vi "align_vi_panel.vi"(8 "error in":errorcluster, 9 "ref vi reference":refnum<vi>, 10 "top vi reference":refnum<vi>, 11 "use top level VI (T)":bool=TRUE) -> (0 "error out":errorcluster)   [LabVIEW 2020, in "varilib.lvlib"]
doc: "LV does not support aligning window to parent window venter. So when this VI is called in the VI with visible panel, it aligns front panel of the caller VI to center of its parent VI front panel or top level VI front panel.\nIn case the top level VI was called asychronously it is necessary to do following:\n1) Call this VI with 'top vi reference' set to reference of the top level VI. This is typically done in main window of application.\n2) Than call this VI within the panel to align with parameter 'use top level VI' set to True. This will use the reference assigned in step 1) as a reference position.\nThis VI also has input 'ref vi reference'. This can be used to set reference position VI directly. It has priority is it is assigned."
uses:
  varilib.lvlib
panel:
  in  "top vi reference memory":refnum<vi>
  out "call chain":string[](array[string])
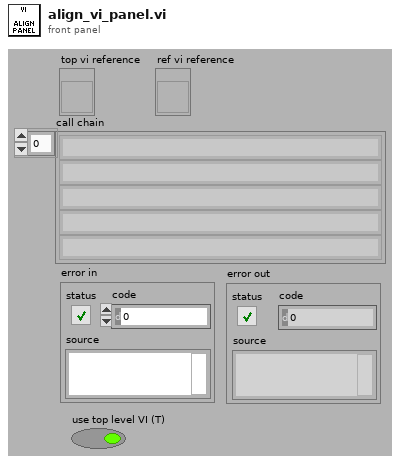
[diagram p1: front panel]
types:
  T1 = typedef "LVRectTypeDef.ctl" = cluster{"Left":i16, "Top":i16, "Right":i16, "Bottom":i16}
  T2 = enum32{"Invalid", "Standard", "Closed", "Hidden", "Minimized", "Maximized"}
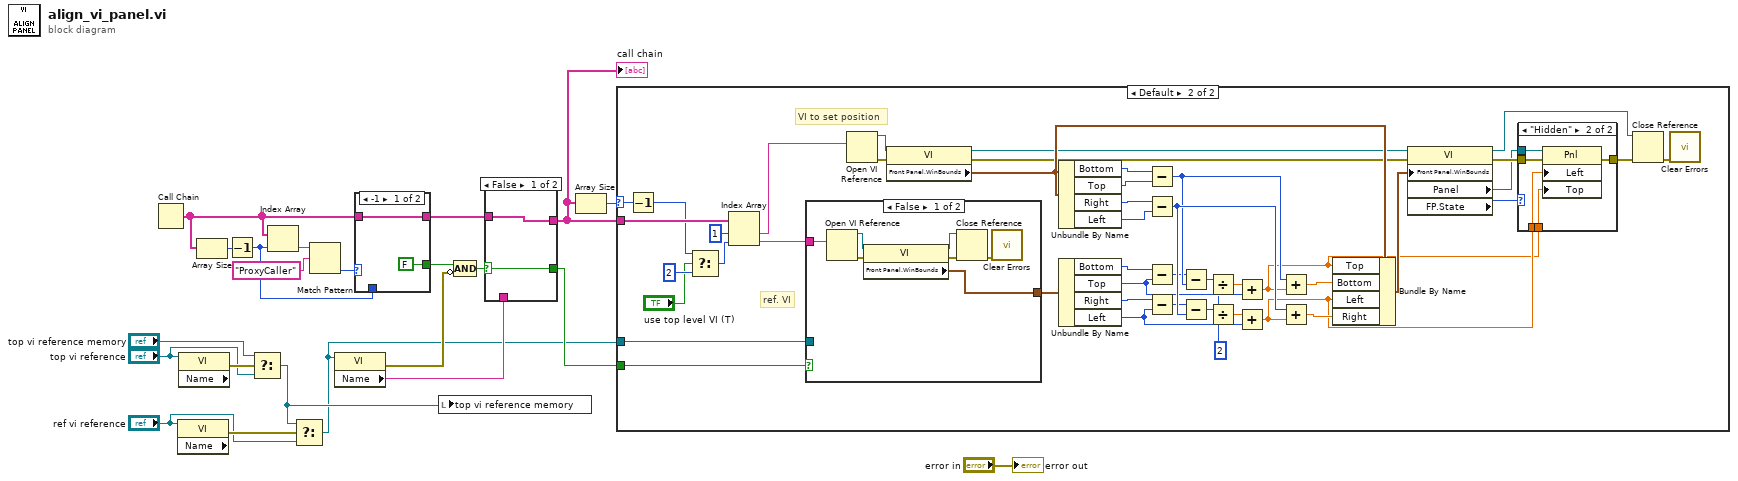
[diagram p0: block diagram]
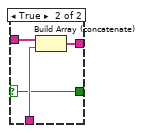
[diagram p2: hidden frame]
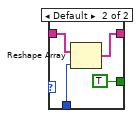
[diagram p3: hidden frame]
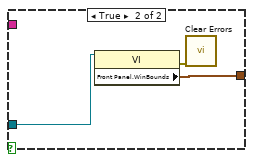
[diagram p6: hidden frame]
diagram:
  n1 = Call Chain() -> (call chain=w17:string[])
  n2 = property class="VI" props=["Name"](reference="ref vi reference") -> (error out=w4:errorcluster)  [unwired: 1 in, 2 out]
  n3 = property class="VI" props=["Name"](reference="top vi reference") -> (error out=w7:errorcluster)  [unwired: 1 in, 2 out]
  n4 = Array Size(array=w17) -> (size(s)=w20:i32)
  n5 = Decrement(x=w20) -> (x-1=w15:i32)
  n6 = Select(t="top vi reference memory", s=w7, f="top vi reference") -> (s? t:f=w2:refnum<vi>)
  n7 = Index Array(array=w17, index=w15) -> (element=w19:string)
  n8 = Select(t=w2, s=w4, f="ref vi reference") -> (s? t:f=w1:refnum<vi>)
  n9 = Match Pattern(string=w19, regular expression="ProxyCaller") -> (offset past match=w16:i32)  [unwired: 1 in, 3 out]
  n10 = property class="VI"(reference=w1) -> (error out=w8:errorcluster, "Name"=w12:string)  [unwired: 1 in, 1 out]
  n11 = case shown="-1" w16 {
    tunnel: w17 -> [w24 w28]
    tunnel: [w24 w27] -> w14
    tunnel: w15 -> [_ w26]
    tunnel: [FALSE TRUE] -> w10
    frame -1 {
    }
    frame Default {
      n12 = Reshape Array(w28, w26) -> (w27:string[])
    }
  }
  n13 = local write "top vi reference memory"(w2) -> ()
  n14 = Compound Arithmetic op=AND(w10, invert w8) -> (w11:bool)
  n15 = case shown="False" w11 {
    selector: w11 -> [w29 w31]
    tunnel: w14 -> [w30 w34]
    tunnel: [w30 w33] -> w13
    tunnel: w12 -> [_ w32]
    tunnel: [w29 w31] -> w9
    frame False {
    }
    frame True {
      n16 = Build Array (concatenate)(w34, w32) -> (w33:string[])
    }
  }
  "call chain" <- w13
  n17 = Array Size(array=w13) -> (size(s)=w21:i32)
  n18 = case shown="Default" w21 {
    selector: w21 -> [_ w48]
    tunnel: w13 -> [_ w51]
    tunnel: w1 -> [_ w43]
    tunnel: w9 -> [_ w42]
    frame 1, 2 {
    }
    frame Default {
      w71 = i16 2 ("y")
      # "ref. VI"
      # "VI to set position"
      n19 = Decrement(x=w48) -> (x-1=w47:i32)
      n20 = Select(t=w47, s="use top level VI (T)", f=2) -> (s? t:f=w49:i32)
      n21 = Index Array(array=w51, index #1=1 ("index"), index #2=w49) -> (element #1=w54:string, element #2=w44:string)
      n22 = case shown="False" w42 {
        tunnel: [w92 w95] -> w53
        tunnel: w44 -> [w86 _]
        tunnel: w43 -> [_ w94]
        frame False {
          n23 = Open VI Reference(vi path=w86) -> (vi reference=w88:refnum<vi>, error out=w89:errorcluster)  [unwired: 5 in]
          n24 = property class="VI"(reference=w88, error in=w89) -> (reference out=w91:refnum<vi>, error out=w90:errorcluster, "Front Panel.WinBounds"=w92:T1)
          n25 = Close Reference(reference=w91, error in (no error)=w90) -> (error out=w87:errorcluster)
          n26 = call <vilib>:"Clear Errors.vi"("error in (no error)"=w87) -> ()  [unwired: 5 in, 2 out]
        }
        frame True {
          n27 = property class="VI"(reference=w94) -> (error out=w93:errorcluster, "Front Panel.WinBounds"=w95:T1)  [unwired: 1 in, 1 out]
          n28 = call <vilib>:"Clear Errors.vi"("error in (no error)"=w93) -> ()  [unwired: 5 in, 2 out]
        }
      }
      n29 = Open VI Reference(vi path=w54) -> (vi reference=w56:refnum<vi>, error out=w55:errorcluster)  [unwired: 5 in]
      n30 = property class="VI"(reference=w56, error in=w55) -> (reference out=w64:refnum<vi>, error out=w63:errorcluster, "Front Panel.WinBounds"=w65:T1)
      n31 = Unbundle By Name(w65) -> ("Bottom"=w69:i16, "Top"=w70:i16, "Right"=w57:i16, "Left"=w73:i16)
      n32 = Unbundle By Name(w53) -> ("Bottom"=w68:i16, "Top"=w76:i16, "Right"=w58:i16, "Left"=w61:i16)
      n33 = Subtract(x=w69, y=w70) -> (x-y=w78:i16)
      n34 = Subtract(x=w57, y=w73) -> (x-y=w79:i16)
      n35 = Subtract(x=w68, y=w76) -> (x-y=w74:i16)
      n36 = Subtract(x=w58, y=w61) -> (x-y=w59:i16)
      n37 = Subtract(x=w74, y=w78) -> (x-y=w75:i16)
      n38 = Subtract(x=w59, y=w79) -> (x-y=w60:i16)
      n39 = Divide(x=w75, y=w71) -> (x/y=w72:dbl)
      n40 = Divide(x=w60, y=w71) -> (x/y=w62:dbl)
      n41 = Add(x=w72, y=w76) -> (x+y=w36:dbl)
      n42 = Add(x=w62, y=w61) -> (x+y=w37:dbl)
      n43 = Add(x=w78, y=w36) -> (x+y=w77:dbl)
      n44 = Add(x=w79, y=w37) -> (x+y=w67:dbl)
      n45 = Bundle By Name(cluster=w65, "Top"=w36, "Bottom"=w77, "Left"=w37, "Right"=w67) -> (w66:T1)
      n46 = property class="VI"(reference=w64, error in=w63, "Front Panel.WinBounds"=w66) -> (reference out=w39:refnum<vi>, error out=w41:errorcluster, "Panel"=w40:refnum<vi>, "FP.State"=w35:T2)
      n47 = case shown="\"Hidden\"" w35 {
        tunnel: w41 -> [w80 w85]
        tunnel: w40 -> [_ w84]
        tunnel: [w80 w83] -> w38
        tunnel: w37 -> [_ w82]
        tunnel: w36 -> [_ w81]
        frame Default {
        }
        frame "Hidden" {
          n48 = property class="Pnl"(reference=w84, error in=w85, "Left"=w82, "Top"=w81) -> (error out=w83:errorcluster)  [unwired: 1 out]
        }
      }
      n49 = Close Reference(reference=w39, error in (no error)=w38) -> (error out=w52:errorcluster)
      n50 = call <vilib>:"Clear Errors.vi"("error in (no error)"=w52) -> ()  [unwired: 5 in, 2 out]
    }
  }
  "error out" <- "error in"
